vi "decodeExt.vi"(8 "error in (no error)":errorcluster, 11 "ByteArray":u8[](array[numeric]) format="%x") -> (0 "error out":errorcluster, 1 "BinaryArray":u8[](array[numeric]), 2 "Variant":variant, 3 "RemainingBytes":u8[](array[numeric]) format="%x", 4 "Ext Type":i8, 5 "Type":string)   [LabVIEW 2015, in "MsgPack.lvlib"]
uses:
  MsgPack.lvlib
  <vilib>/ErrorRing/Error Ring.xnode
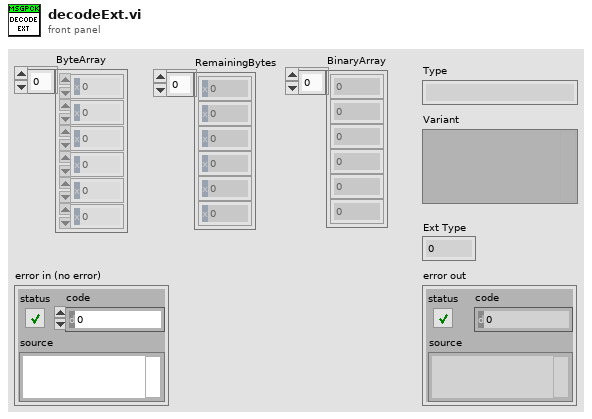
[diagram p1: front panel]
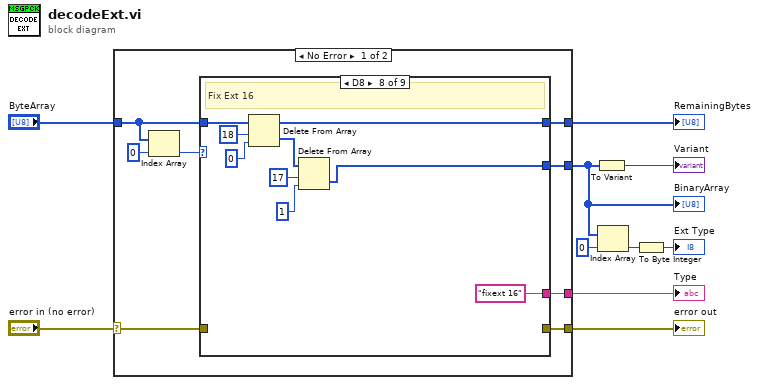
[diagram p0: block diagram]
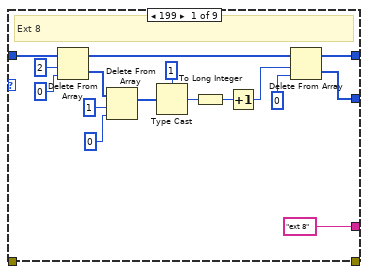
[diagram p2: hidden frame]
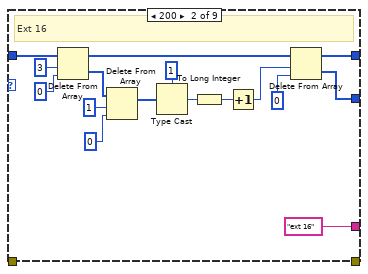
[diagram p3: hidden frame]
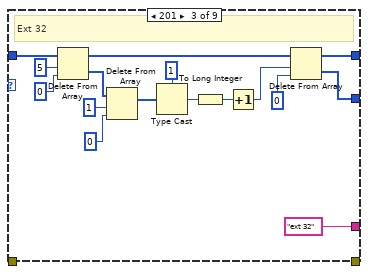
[diagram p4: hidden frame]
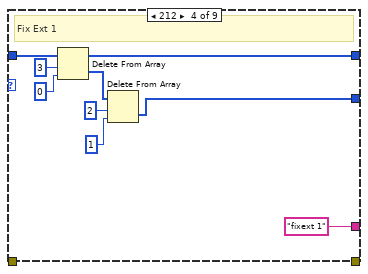
[diagram p5: hidden frame]
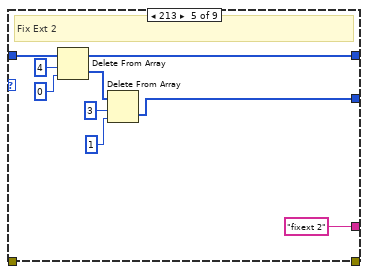
[diagram p6: hidden frame]
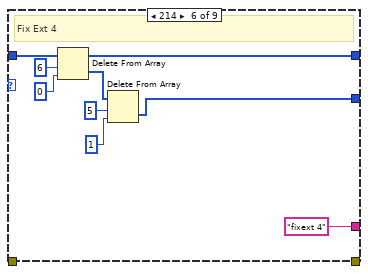
[diagram p7: hidden frame]
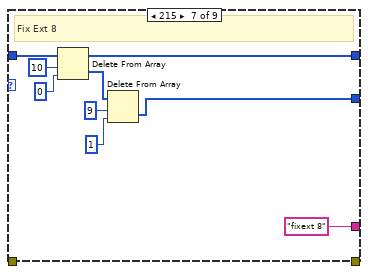
[diagram p8: hidden frame]
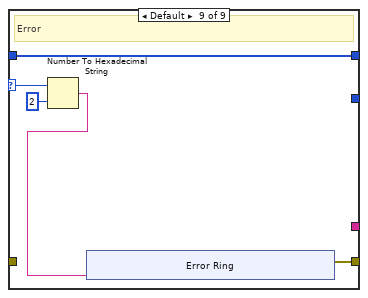
[diagram p9: hidden frame]
diagram:
  n1 = case shown="No Error" "error in (no error)" {
    selector: "error in (no error)" -> [w15 w123]
    tunnel: [w18 w123] -> w9
    tunnel: [w17 _] -> w8
    tunnel: [w16 _] -> w4
    tunnel: "ByteArray" -> [w13 w122]
    tunnel: [w14 w122] -> w6
    frame No Error {
      n2 = Index Array(array=w13, index=0) -> (element=w12:u8)
      n3 = case shown="D8" w12 {
        selector: w12 -> [_ _ _ _ _ _ _ _ w113]
        tunnel: [_ _ _ _ _ _ _ _ w115] -> w18
        tunnel: w15 -> [_ _ _ _ _ _ _ _ _]
        tunnel: ["ext 8" "ext 16" "ext 32" "fixext 1" "fixext 2" "fixext 4" "fixext 8" "fixext 16" _] -> w17
        tunnel: [w22 w38 w54 w67 w76 w85 w94 w103 _] -> w16
        tunnel: [w27 w43 w59 w68 w77 w86 w95 w104 w116] -> w14
        tunnel: w13 -> [w32 w48 w64 w73 w82 w91 w100 w109 w116]
        frame 199 {
          # "Ext 8"
          n4 = Delete From Array(array=w32, length=2, index=0) -> (deleted portion=w26:u8[], array with subset deleted=w28:u8[])
          n5 = Delete From Array(array=w26, length=1, index=0) -> (array with subset deleted=w25:u8[])  [unwired: 1 out]
          n6 = Type Cast(type=u8 1 ("index"), x=w25) -> (*(type *) &x=w20:u8)
          n7 = To Long Integer(number=w20) -> (32bit integer=w19:i32)
          n8 = Increment(x=w19) -> (x+1=w21:i32)
          n9 = Delete From Array(array=w28, length=w21, index=0) -> (deleted portion=w22:u8[], array with subset deleted=w27:u8[])
        }
        frame 200 {
          # "Ext 16"
          n10 = Delete From Array(array=w48, length=3, index=0) -> (deleted portion=w42:u8[], array with subset deleted=w44:u8[])
          n11 = Delete From Array(array=w42, length=1, index=0) -> (array with subset deleted=w41:u8[])  [unwired: 1 out]
          n12 = Type Cast(type=u16 1 ("index"), x=w41) -> (*(type *) &x=w36:u16)
          n13 = To Long Integer(number=w36) -> (32bit integer=w35:i32)
          n14 = Increment(x=w35) -> (x+1=w37:i32)
          n15 = Delete From Array(array=w44, length=w37, index=0) -> (deleted portion=w38:u8[], array with subset deleted=w43:u8[])
        }
        frame 201 {
          # "Ext 32"
          n16 = Delete From Array(array=w64, length=5, index=0) -> (deleted portion=w58:u8[], array with subset deleted=w60:u8[])
          n17 = Delete From Array(array=w58, length=1, index=0) -> (array with subset deleted=w57:u8[])  [unwired: 1 out]
          n18 = Type Cast(type=u32 1 ("index"), x=w57) -> (*(type *) &x=w52:u32)
          n19 = To Long Integer(number=w52) -> (32bit integer=w51:i32)
          n20 = Increment(x=w51) -> (x+1=w53:i32)
          n21 = Delete From Array(array=w60, length=w53, index=0) -> (deleted portion=w54:u8[], array with subset deleted=w59:u8[])
        }
        frame 212 {
          # "Fix Ext 1"
          n22 = Delete From Array(array=w73, length=3, index=0) -> (deleted portion=w71:u8[], array with subset deleted=w68:u8[])
          n23 = Delete From Array(array=w71, length=2, index=1) -> (deleted portion=w67:u8[])  [unwired: 1 out]
        }
        frame 213 {
          # "Fix Ext 2"
          n24 = Delete From Array(array=w82, length=4, index=0) -> (deleted portion=w80:u8[], array with subset deleted=w77:u8[])
          n25 = Delete From Array(array=w80, length=3, index=1) -> (deleted portion=w76:u8[])  [unwired: 1 out]
        }
        frame 214 {
          # "Fix Ext 4"
          n26 = Delete From Array(array=w91, length=6, index=0) -> (deleted portion=w89:u8[], array with subset deleted=w86:u8[])
          n27 = Delete From Array(array=w89, length=5, index=1) -> (deleted portion=w85:u8[])  [unwired: 1 out]
        }
        frame 215 {
          # "Fix Ext 8"
          n28 = Delete From Array(array=w100, length=10, index=0) -> (deleted portion=w98:u8[], array with subset deleted=w95:u8[])
          n29 = Delete From Array(array=w98, length=9, index=1) -> (deleted portion=w94:u8[])  [unwired: 1 out]
        }
        frame 216 {
          # "Fix Ext 16"
          n30 = Delete From Array(array=w109, length=18, index=0) -> (deleted portion=w107:u8[], array with subset deleted=w104:u8[])
          n31 = Delete From Array(array=w107, length=17, index=1) -> (deleted portion=w103:u8[])  [unwired: 1 out]
        }
        frame Default {
          # "Error"
          n32 = Number To Hexadecimal String(1:i16 2 ("width (-)"), 2:w113) -> (0:w112:string)
          n33 = xnode "Error Ring"("parameter 0"=w112) -> ("error out"=w115:errorcluster)
        }
      }
    }
    frame Error {
    }
  }
  "error out" <- w9
  "Type" <- w8
  "BinaryArray" <- w4
  "RemainingBytes" <- w6
  n34 = To Variant(anything=w4) -> (Variant=→"Variant":variant)
  n35 = Index Array(array=w4, index=0) -> (element=w2:u8)
  n36 = To Byte Integer(number=w2) -> (8bit integer=→"Ext Type":i8)
